vi "DigiPAC_COM_Stop(SubVI).vi"(8 "error in (no error)":errorcluster, 9 "UART Channel (0)":u8, 10 "Detector input":string, 11 "LINX Resource in":T1) -> (0 "error out":errorcluster, 2 "Measurement started?":bool, 3 "LINX Resource out":T1)   [LabVIEW 2017]
uses:
  <vilib>/MakerHub/LINX/Private/Type Defs/LINX Ref.ctl
  <vilib>/MakerHub/LINX/Private/Type Defs/Platform.ctl
  <vilib>/MakerHub/LINX/Private/Type Defs/Interface.ctl
  <vilib>/MakerHub/LINX/Private/Device/Type Defs/LINX Device Config.ctl
  <vilib>/MakerHub/LINX/Private/Device/Type Defs/TCP Config.ctl
  <vilib>/MakerHub/LINX/Private/Device/Type Defs/Channels.ctl
  <vilib>/MakerHub/LINX/Public/Peripherals/UART/UART Write String.vi
  <vilib>/MakerHub/LINX/Public/Peripherals/UART/UART Write Byte Array.vi
  <vilib>/MakerHub/LINX/Private/Local IO/LinxUartWrite.vi
  <vilib>/MakerHub/LINX/Public/Utilities/Check Channel.vi
  <vilib>/MakerHub/LINX/Private/Utilties/Generate Error.vi
  <vilib>/MakerHub/LINX/Public/Peripherals/UART/UART Read String.vi
  <vilib>/MakerHub/LINX/LMH-LINX.lvlib
  <vilib>/MakerHub/LINX/Private/Device/Device.lvlib
panel:
  out "Confirmation message":string
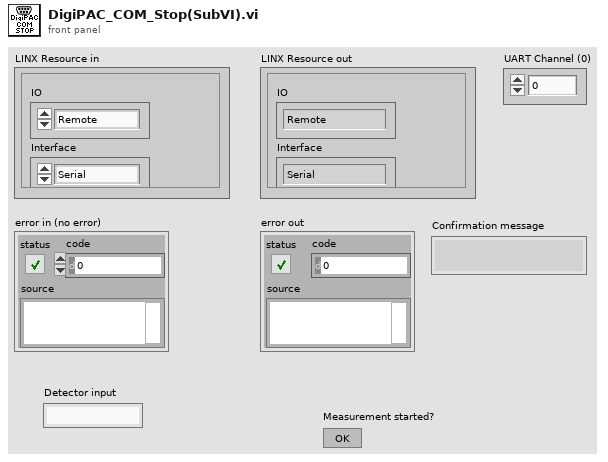
[diagram p1: front panel]
types:
  T1 = typedef "LMH-LINX.lvlib/LINX Ref.ctl" = cluster{"IO":T2, "Interface":T3, "LINX Device Config":T4}
  T2 = typedef "LMH-LINX.lvlib/Platform.ctl" = enum16{"Remote", "Local"}
  T3 = typedef "LMH-LINX.lvlib/Interface.ctl" = enum16{"Serial", "TCP"}
  T4 = typedef "LMH-LINX.lvlib/Device.lvlib/LINX Device Config.ctl" = cluster{"Interface":T3, "COM Port":refnum<visa-resource-name>, "TCP Configuration":T5, "Device Family":u8, "Device ID":u8, "Device Name":string, "TCP Ref":refnum<k5>, "Channels":T6}
  T5 = typedef "LMH-LINX.lvlib/Device.lvlib/TCP Config.ctl" = cluster{"IP Address":string, "Port":u16}
  T6 = typedef "LMH-LINX.lvlib/Channels.ctl" = cluster{"DI":u8[], "DO":u8[], "AI":u8[], "AO":u8[], "PWM":u8[], "QE":u8[], "UART":u8[], "I2C 2":u8[], "SPI":u8[], "CAN":u8[], "Servo":u8[], "AI Ref (V)":dbl, "AI Resolution (Bits)":u8, "AO Ref (V)":dbl, "AO Resolution (Bits)":u8}
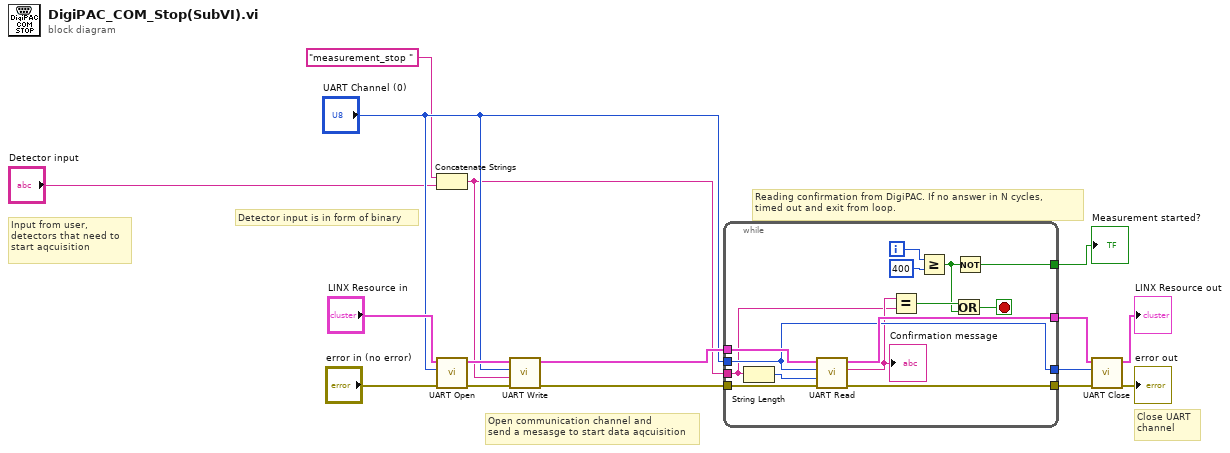
[diagram p0: block diagram]
diagram:
  # "Detector input is in form of binary"
  # "Input from user,\ndetectors that need to \nstart aqcuisition"
  # "Close UART\nchannel"
  # "Open communication channel and \nsend a mesasge to start data aqcuisition"
  # "Reading confirmation from DigiPAC. If no answer in N cycles, \ntimed out and exit from loop."
  n1 = Concatenate Strings("measurement_stop " ("Data"), "Detector input") -> (w1:string)
  n2 = call <vilib>:"UART Open.vi"("Error In"="error in (no error)", "UART Channel (0)"="UART Channel (0)", "LINX Resource"="LINX Resource in") -> ("Error Out"=w13:errorcluster, "LINX Resource"=w14:T1)  [unwired: 6 in, 1 out]
  n3 = call-poly <vilib>:"UART Write.vi"("Error In"=w13, "Data"=w1, "UART Channel (0)"="UART Channel (0)", "LINX Resource"=w14) -> ("Error Out"=w11:errorcluster, "LINX Resource"=w12:T1)  [unwired: 6 in]
  n4 = while {
    tunnel: w12 -> [w30]
    tunnel: w11 -> [w29]
    tunnel: [w28] -> w10
    tunnel: [w27] -> w9
    tunnel: "UART Channel (0)" -> [w26]
    tunnel: [w26] -> w8
    tunnel: [w18] -> w2
    tunnel: w1 -> [w17]
    i -> [w24]
    stop <- w20 stop-if-true
    n5 = String Length(string=w17) -> (length=w25:i32)
    n6 = call-poly <vilib>:"UART Read.vi"("Error In"=w29, "Num Bytes"=w25, "UART Channel (0)"=w26, "LINX Resource"=w30) -> ("Error Out"=w27:errorcluster, "Data"=w21:string, "LINX Resource"=w28:T1)  [unwired: 5 in]
    "Confirmation message" <- w21
    n7 = Equal?(x=w21, y=w17) -> (x = y?=w22:bool)
    n8 = Greater Or Equal?(x=w24, y=400) -> (x >= y?=w19:bool)
    n9 = Or(x=w22, y=w19) -> (x .or. y?=w20:bool)
    n10 = Not(x=w19) -> (.not. x?=w18:bool)
  }
  "Measurement started?" <- w2
  n11 = call <vilib>:"UART Close.vi"("Error In"=w9, "UART Channel (0)"=w8, "LINX Resource"=w10) -> ("Error Out"=→"error out":errorcluster, "LINX Resource"=→"LINX Resource out":T1)  [unwired: 7 in]
